vi "read_TCUStatus1.vi"(11 "Message":u8[](array[numeric])) -> (3 "Status1":T1)   [LabVIEW 2017]
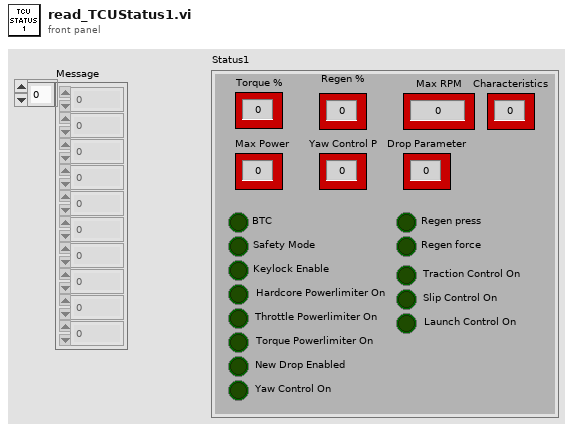
[diagram p1: front panel]
types:
  T1 = cluster{"Regen %":u8, "Characteristics":u8, "Drop Parameter":dbl, "Yaw Control P":u16, "Max Power":u8, "Torque %":u8, "Max RPM":u16, "Regen press":bool, "Regen force":bool, "BTC":bool, "Safety Mode":bool, "Keylock Enable":bool, "Hardcore Powerlimiter On":bool, "Throttle Powerlimiter On":bool, "Torque Powerlimiter On":bool, "New Drop Enabled":bool, "Yaw Control On":bool, "Traction Control On":bool, "Slip Control On":bool, "Launch Control On":bool}
  T2 = cluster{"Regen %":u8, "Characteristics":u8, "Drop Parameter":dbl, "Yaw Control P":u16, "Max Power":u8, "Torque %":u8, "Max RPM":u16, "Regen force":bool, "Regen press":bool, "BTC":bool, "Safety Mode":bool, "Keylock Enable":bool, "Hardcore Powerlimiter On":bool, "Throttle Powerlimiter On":bool, "Torque Powerlimiter On":bool, "New Drop Enabled":bool, "Yaw Control On":bool, "Traction Control On":bool, "Slip Control On":bool, "Launch Control On":bool}
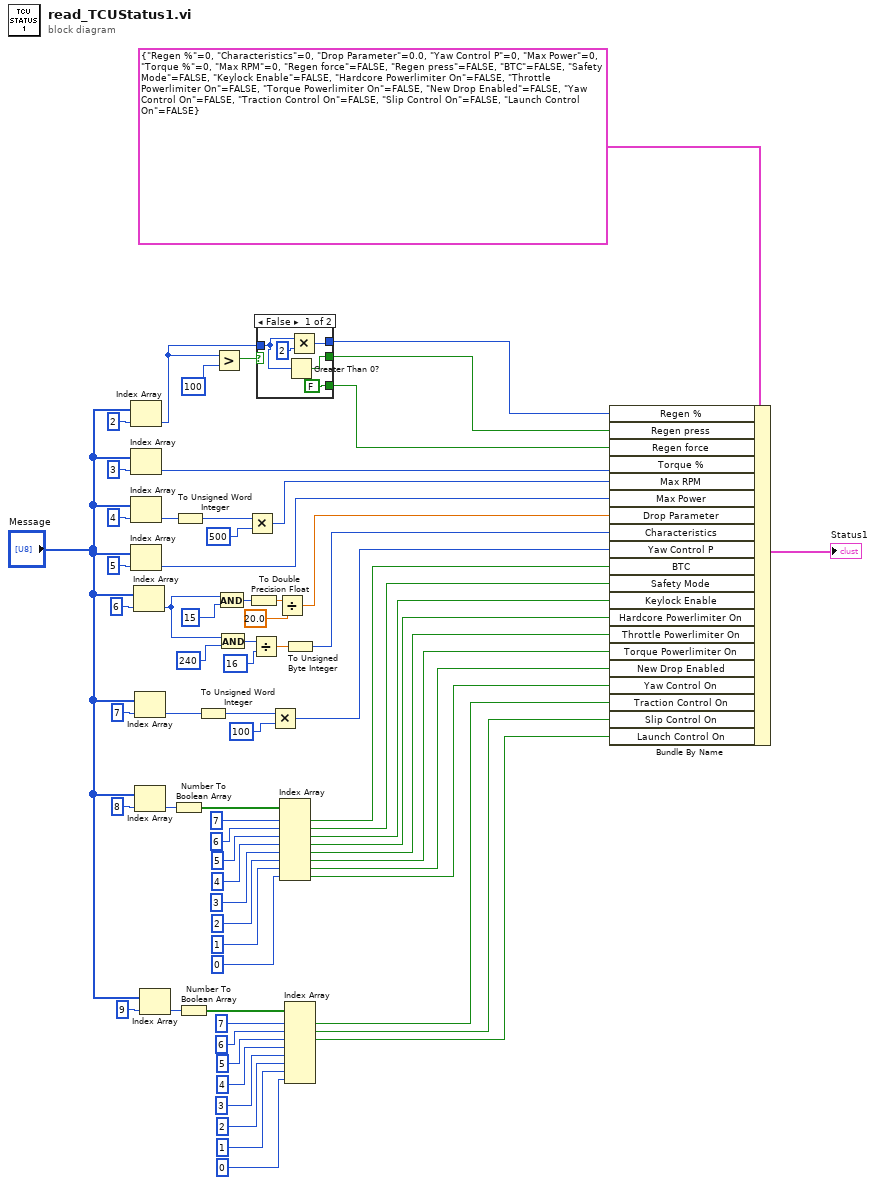
[diagram p0: block diagram]
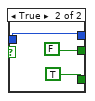
[diagram p2: hidden frame]
diagram:
  n1 = Index Array(array="Message", index=2) -> (element=w53:u8)
  n2 = Index Array(array="Message", index=3) -> (element=w60:u8)
  n3 = Index Array(array="Message", index=4) -> (element=w59:u8)
  n4 = Index Array(array="Message", index=5) -> (element=w55:u8)
  n5 = Index Array(array="Message", index=6) -> (element=w48:u8)
  n6 = Index Array(array="Message", index=7) -> (element=w6:u8)
  n7 = Index Array(array="Message", index=8) -> (element=w41:u8)
  n8 = Index Array(array="Message", index=9) -> (element=w14:u8)
  n9 = Number To Boolean Array(number=w41) -> (Boolean array=w40:bool[])
  n10 = To Unsigned Word Integer(number=w59) -> (unsigned 16bit integer=w57:u16)
  n11 = Number To Boolean Array(number=w14) -> (Boolean array=w15:bool[])
  n12 = To Unsigned Word Integer(number=w6) -> (unsigned 16bit integer=w8:u16)
  n13 = Greater?(x=w53, y=u8 100) -> (0:w52:bool)
  n14 = And(x=w48, y=u8 15) -> (x .and. y?=w4:u8)
  n15 = And(x=w48, y=u8 240) -> (x .and. y?=w45:u8)
  n16 = Multiply(x=w57, y=u16 500) -> (x*y=w56:u16)
  n17 = To Double Precision Float(number=w4) -> (double precision float=w3:dbl)
  n18 = Divide(x=w45, y=u8 16) -> (x/y=w43:dbl)
  n19 = case shown="False" w52 {
    tunnel: [w74 w77] -> w51
    tunnel: w53 -> [w70 w77]
    tunnel: [w72 FALSE] -> w50
    tunnel: [FALSE TRUE] -> w49
    frame False {
      n20 = Greater Than 0?(x=w70) -> (x > 0?=w72:bool)
      n21 = Multiply(x=w70, y=u8 2) -> (x*y=w74:u8)
    }
    frame True {
    }
  }
  n22 = Multiply(x=w8, y=u16 100) -> (x*y=w5:u16)
  n23 = Divide(x=w3, y=20.0) -> (x/y=w2:dbl)
  n24 = Index Array(array=w40, index #1=7 ("index"), index #2=6 ("index"), index #3=5 ("index"), index #4=4 ("index"), index #5=3 ("index"), index #6=2 ("index"), index #7=1 ("index"), index #8=0 ("index")) -> (element #1=w36:bool, element #2=w35:bool, element #3=w34:bool, element #4=w33:bool, element #5=w27:bool, element #6=w26:bool, element #7=w25:bool, element #8=w24:bool)
  n25 = To Unsigned Byte Integer(number=w43) -> (unsigned 8bit integer=w42:u8)
  n26 = Index Array(array=w15, index #1=7 ("index"), index #2=6 ("index"), index #3=5 ("index"), index #4=4 ("index"), index #5=3 ("index"), index #6=2 ("index"), index #7=1 ("index"), index #8=0 ("index")) -> (element #1=w11:bool, element #2=w10:bool, element #3=w9:bool)  [unwired: 5 out]
  n27 = Bundle By Name(cluster=T2 {"Regen %"=0, "Characteristics"=0, "Drop Parameter"=0.0, "Yaw Control P"=0, "Max Power"=0, "Torque %"=0, "Max RPM"=0, "Regen force"=FALSE, "Regen press"=FALSE, "BTC"=FALSE, "Safety Mode"=FALSE, "Keylock Enable"=FALSE, "Hardcore Powerlimiter On"=FALSE, "Throttle Powerlimiter On"=FALSE, "Torque Powerlimiter On"=FALSE, "New Drop Enabled"=FALSE, "Yaw Control On"=FALSE, "Traction Control On"=FALSE, "Slip Control On"=FALSE, "Launch Control On"=FALSE} ("Cluster"), "Regen %"=w51, "Regen press"=w50, "Regen force"=w49, "Torque %"=w60, "Max RPM"=w56, "Max Power"=w55, "Drop Parameter"=w2, "Characteristics"=w42, "Yaw Control P"=w5, "BTC"=w36, "Safety Mode"=w35, "Keylock Enable"=w34, "Hardcore Powerlimiter On"=w33, "Throttle Powerlimiter On"=w27, "Torque Powerlimiter On"=w26, "New Drop Enabled"=w25, "Yaw Control On"=w24, "Traction Control On"=w11, "Slip Control On"=w10, "Launch Control On"=w9) -> (→"Status1":T2)
